vi "EnemyKick.vi"(6 "atacando contra?":bool, 9 "balls":T1[](array[typedef]), 10 "Field Size in":T5, 11 "Robot in":T2={"id"=0, "function"=enum."Attacker", "x"=0.0, "y"=0.0, "orientation"=0.0, "v_tangent"=0.0, "v_normal"=0.0, "v_ang"=0.0, "kick_x"=0.0, "kick_z"=0.0, "dribble"=FALSE, "Timestamp"=timestamp(0 s since 1904-01-01), "dest_x"=0.0, "dest_y"=0.0, "dest_orientation"=0.0, "estimatives"={"est_v_tangent"=0.0, "est_v_normal"=0.0, "est_vx"=0.0, "est_vy"=0.0}, "dest_x_kick"=0.0, "dest_y_kick"=0.0, "Gap Coord"=[], "States"=enum."GoToTangent"}) -> (3 "Robot out":T2={"id"=0, "function"=enum."Attacker", "x"=0.0, "y"=0.0, "orientation"=0.0, "v_tangent"=0.0, "v_normal"=0.0, "v_ang"=0.0, "kick_x"=0.0, "kick_z"=0.0, "dribble"=FALSE, "Timestamp"=timestamp(0 s since 1904-01-01), "dest_x"=0.0, "dest_y"=0.0, "dest_orientation"=0.0, "estimatives"={"est_v_tangent"=0.0, "est_v_normal"=0.0, "est_vx"=0.0, "est_vy"=0.0}, "dest_x_kick"=0.0, "dest_y_kick"=0.0, "Gap Coord"=[], "States"=enum."GoToTangent"})   [LabVIEW 2016]
uses:
  Core/Field Size.ctl
  Core/AI Robot.ctl
  Functions Enum.ctl
  AttackerStates.ctl
  Core/AI Ball.ctl
  <vilib>/Analysis/_algsub.llb/Real Vector Norm.vi
  <vilib>/Analysis/NI_AALPro.lvlib
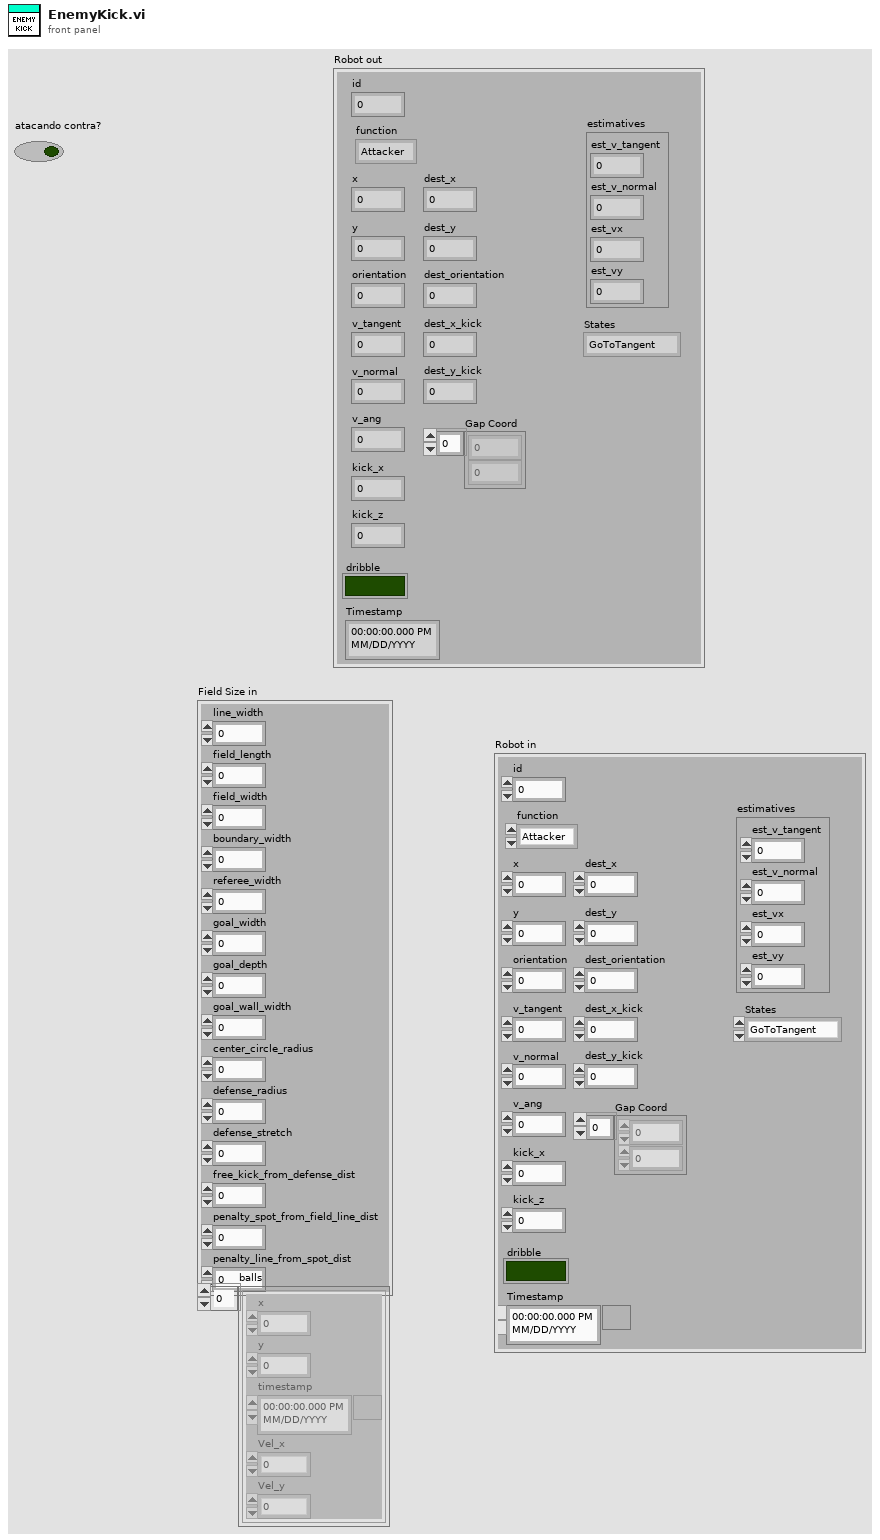
[diagram p1: front panel]
types:
  T1 = typedef "AI Ball.ctl" = cluster{"x":dbl, "y":dbl, "timestamp":timestamp, "Vel_x":dbl, "Vel_y":dbl}
  T2 = typedef "AI Robot.ctl" = cluster{"id":u32, "function":T3, "x":dbl, "y":dbl, "orientation":dbl, "v_tangent":dbl, "v_normal":dbl, "v_ang":dbl, "kick_x":dbl, "kick_z":dbl, "dribble":bool, "Timestamp":timestamp, "dest_x":dbl, "dest_y":dbl, "dest_orientation":dbl, "estimatives":cluster{"est_v_tangent":dbl, "est_v_normal":dbl, "est_vx":dbl, "est_vy":dbl}, "dest_x_kick":dbl, "dest_y_kick":dbl, "Gap Coord":dbl[], "States":T4}
  T3 = typedef "Functions Enum.ctl" = enum16{"Attacker", "Goalie", "Defender", "Striker", "Goto 0", "Dummy", "Kicker", "ZigZag"}
  T4 = typedef "AttackerStates.ctl" = enum16{"Pass", "GoToTangent", "BallGetting", "GoToKick", ""}
  T5 = typedef "Field Size.ctl" = cluster{"line_width":u32, "field_length":u32, "field_width":u32, "boundary_width":u32, "referee_width":u32, "goal_width":u32, "goal_depth":u32, "goal_wall_width":u32, "center_circle_radius":u32, "defense_radius":u32, "defense_stretch":u32, "free_kick_from_defense_dist":u32, "penalty_spot_from_field_line_dist":u32, "penalty_line_from_spot_dist":u32}
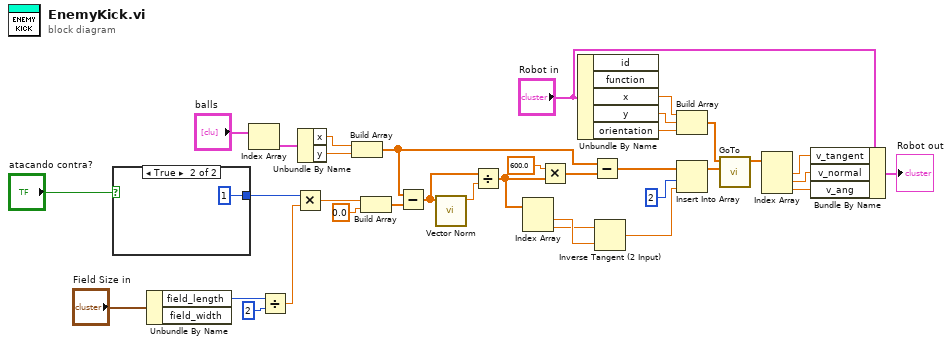
[diagram p0: block diagram]
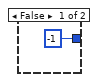
[diagram p2: hidden frame]
diagram:
  n1 = case shown="True" "atacando contra?" {
    tunnel: [-1 1] -> w14
    frame False {
    }
    frame True {
    }
  }
  n2 = Unbundle By Name("Field Size in") -> ("field_length"=w34:u32)  [unwired: 1 out]
  n3 = Index Array(array="balls") -> (element=w30:T1)  [unwired: 1 in]
  n4 = Divide(x=w34, y=u32 2) -> (x/y=w25:dbl)
  n5 = Multiply(x=w14, y=w25) -> (x*y=w13:dbl)
  n6 = Unbundle By Name(w30) -> ("x"=w32:dbl, "y"=w31:dbl)
  n7 = Build Array(w32, w31) -> (w15:dbl[])
  n8 = Build Array(w13, 0.0 ("element")) -> (w9:dbl[])
  n9 = Subtract(x=w15, y=w9) -> (x-y=w10:dbl[])
  n10 = call-poly <vilib>:"Vector Norm.vi"("Input Vector"=w10) -> ("norm"=w11:dbl)  [unwired: 9 in, 1 out]
  n11 = Divide(x=w10, y=w11) -> (x/y=w4:dbl[])
  n12 = Index Array(array=w4) -> (element #1=w6:dbl, element #2=w5:dbl)  [unwired: 2 in]
  n13 = Multiply(x=600.0, y=w4) -> (x*y=w2:dbl[])
  n14 = Unbundle By Name("Robot in") -> ("x"=w29:dbl, "y"=w28:dbl, "orientation"=w27:dbl)  [unwired: 2 out]
  n15 = Subtract(x=w15, y=w2) -> (x-y=w1:dbl[])
  n16 = Inverse Tangent (2 Input)(1:w6, 2:w5) -> (0:w7:dbl)
  n17 = Build Array(w29, w28, w27) -> (w17:dbl[])
  n18 = Insert Into Array(array=w1, index=2, new element=w7) -> (w16:dbl[])
  n19 = call "GoTo.vi"("Target"=w16, "Position"=w17) -> ("Output\nVelocity"=w19:dbl[])  [unwired: 8 in, 1 out]
  n20 = Index Array(array=w19) -> (element #1=w22:dbl, element #2=w23:dbl, element #3=w24:dbl)  [unwired: 3 in]
  n21 = Bundle By Name(cluster="Robot in", "v_tangent"=w22, "v_normal"=w23, "v_ang"=w24) -> (→"Robot out":T2)
